vi "absolute_position.vi"(6 "Encoder rotates cw":bool, 7 "curr. angle":dbl format="%#_13g", 8 "Absolute position in":dbl=-1.0, 11 "prev. angle":dbl format="%#_13g") -> (0 "Absolute position out":dbl, 1 "relative position wheel":dbl, 2 "relative position shaft":dbl, 3 "Wheel Position (abs)":dbl)   [LabVIEW 2019]
panel:
  out "angular difference":dbl
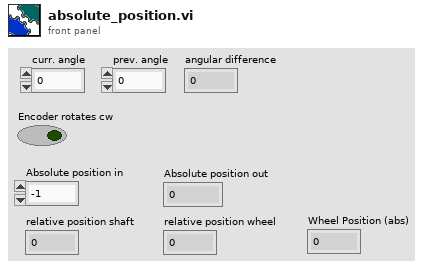
[diagram p1: front panel]
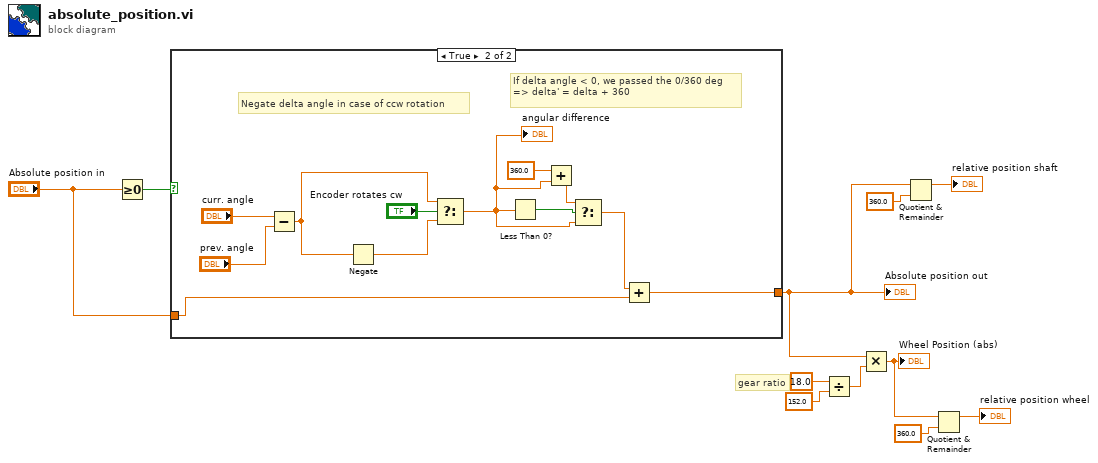
[diagram p0: block diagram]
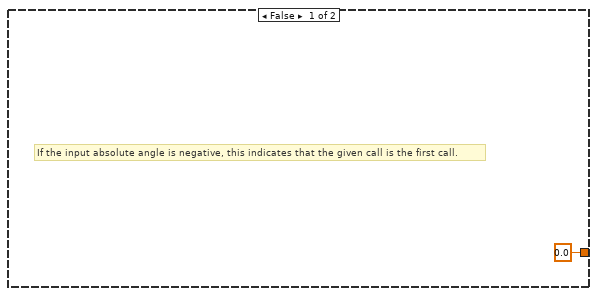
[diagram p2: hidden frame]
diagram:
  # "gear ratio"
  n1 = Greater Or Equal To 0?(x="Absolute position in") -> (x >= 0?=w8:bool)
  n2 = case shown="True" w8 {
    tunnel: "Absolute position in" -> [_ w16]
    tunnel: [0.0 w15] -> w5
    frame False {
      # "If the input absolute angle is negative, this indicates that the given call is the first call."
    }
    frame True {
      # "If delta angle < 0, we passed the 0/360 deg => delta' = delta + 360"
      # "Negate delta angle in case of ccw rotation"
      n3 = Subtract(x="curr. angle", y="prev. angle") -> (x-y=w14:dbl)
      n4 = Negate(x=w14) -> (-x=w13:dbl)
      n5 = Select(t=w14, s="Encoder rotates cw", f=w13) -> (s? t:f=w18:dbl)
      "angular difference" <- w18
      n6 = Less Than 0?(x=w18) -> (x < 0?=w21:bool)
      n7 = Add(x=360.0, y=w18) -> (x+y=w19:dbl)
      n8 = Select(t=w19, s=w21, f=w18) -> (s? t:f=w17:dbl)
      n9 = Add(x=w17, y=w16) -> (x+y=w15:dbl)
    }
  }
  "Absolute position out" <- w5
  n10 = Divide(x=18.0, y=152.0) -> (x/y=w9:dbl)
  n11 = Multiply(x=w5, y=w9) -> (x*y=w1:dbl)
  "Wheel Position (abs)" <- w1
  n12 = Quotient & Remainder(x=w5, y=360.0) -> (x-y*floor(x/y)=→"relative position shaft":dbl)  [unwired: 1 out]
  n13 = Quotient & Remainder(x=w1, y=360.0) -> (x-y*floor(x/y)=→"relative position wheel":dbl)  [unwired: 1 out]
